vi "Read_Env.vi"(0 "COM Bluegiga in":refnum<visa-resource-name>, 2 "Handle table":string[][](array[string]), 5 "Characteristic UUID":string, 6 "Service UUID":string, 7 "error in (no error)":errorcluster, 15 "Connection Status":T1={"MAC Address"="", "cnx handle"=0, "cnx flags"=0, "Address Type"=125, "Connection Interval (ms)"=125, "Timeout(ms)"=125, "Latency"=0, "bonding handle"=0} {"Address Type" items=["Public", "Random"]}) -> (8 "Intervalo Temperatura":u16, 9 "Intensidad Verde":u8, 10 "Intervalo Humedad":u16, 11 "Intensidad Azul":u8, 12 "Intervalo Presion":u16, 14 "Intervalo Color":u16, 16 "Modo Aire":u8, 18 "Intensidad Rojo":u8, 20 "COM Bluegiga out":refnum<visa-resource-name>, 23 "Registro Completo":u8[](array[numeric]), 27 "error out":errorcluster)   [LabVIEW 2020]
uses:
  <vilib>/BLE/type_def/connection_status_bundle.ctl
  <vilib>/BLE/type_def/address_type.ctl
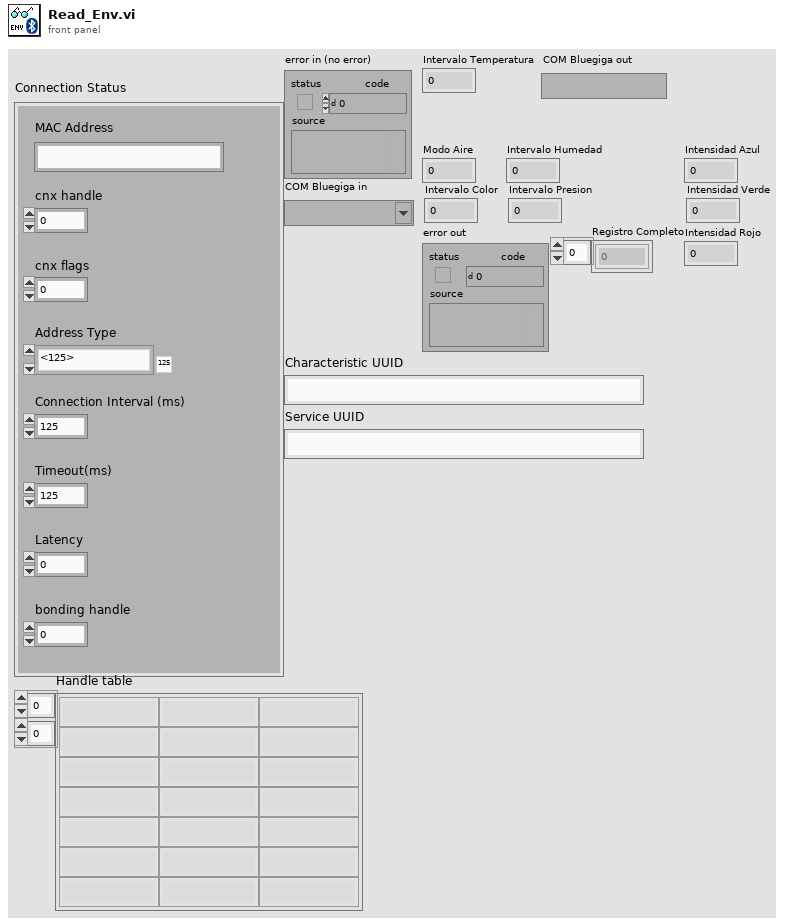
[diagram p1: front panel]
types:
  T1 = typedef "connection_status_bundle.ctl" = cluster{"MAC Address":string, "cnx handle":u8, "cnx flags":u8, "Address Type":T2, "Connection Interval (ms)":u16, "Timeout(ms)":u16, "Latency":u16, "bonding handle":u8}
  T2 = typedef "address_type.ctl" = u8
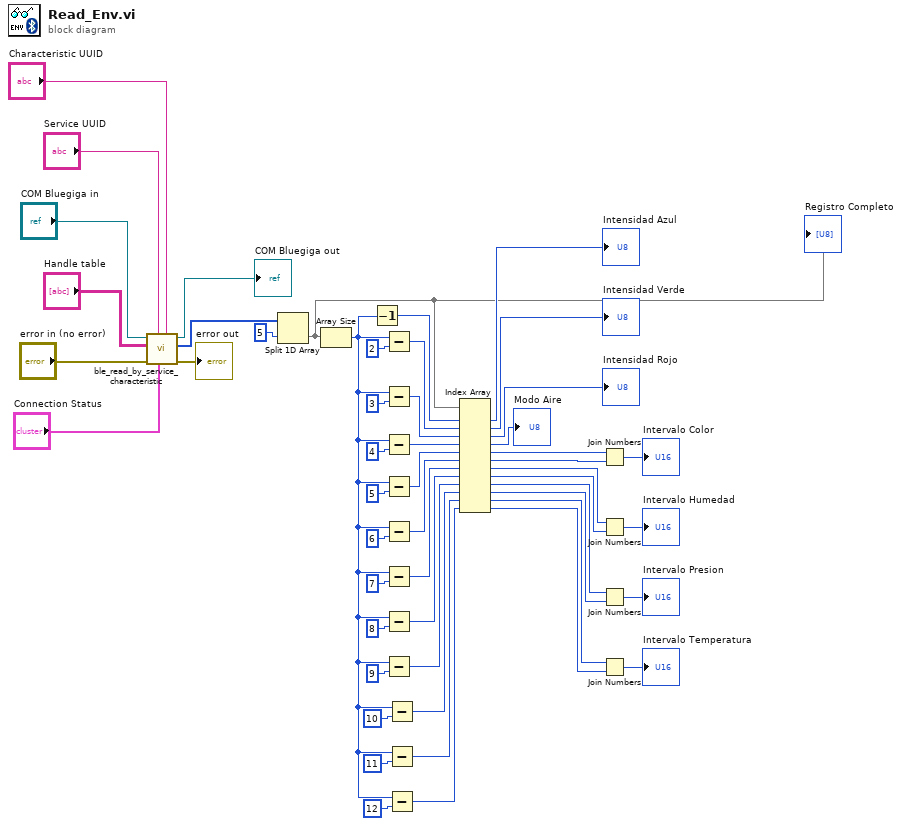
[diagram p0: block diagram]
diagram:
  n1 = call <vilib>:"ble_read_by_service_characteristic.vi"("Characteristic UUID"="Characteristic UUID", "Connection Status"="Connection Status", "Service UUID"="Service UUID", "error in (no error)"="error in (no error)", "Handle table"="Handle table", "COM Bluegiga in"="COM Bluegiga in") -> ("error out"=→"error out":errorcluster, "characteristic value"=w9:u8[], "COM Bluegiga out"=→"COM Bluegiga out":refnum<visa-resource-name>)  [unwired: 3 in]
  n2 = Split 1D Array(array=w9, index=5) -> (second subarray=w11:u8[])  [unwired: 1 out]
  "Registro Completo" <- w11
  n3 = Array Size(array=w11) -> (size(s)=w41:i32)
  n4 = Decrement(x=w41) -> (x-1=w51:i32)
  n5 = Subtract(x=w41, y=2) -> (x-y=w50:i32)
  n6 = Subtract(x=w41, y=3) -> (x-y=w49:i32)
  n7 = Subtract(x=w41, y=4) -> (x-y=w48:i32)
  n8 = Subtract(x=w41, y=5) -> (x-y=w47:i32)
  n9 = Subtract(x=w41, y=6) -> (x-y=w46:i32)
  n10 = Subtract(x=w41, y=7) -> (x-y=w45:i32)
  n11 = Subtract(x=w41, y=8) -> (x-y=w44:i32)
  n12 = Subtract(x=w41, y=9) -> (x-y=w43:i32)
  n13 = Subtract(x=w41, y=10) -> (x-y=w42:i32)
  n14 = Subtract(x=w41, y=11) -> (x-y=w40:i32)
  n15 = Subtract(x=w41, y=12) -> (x-y=w39:i32)
  n16 = Index Array(array=w11, index #1=w51, index #2=w50, index #3=w49, index #4=w48, index #5=w47, index #6=w46, index #7=w45, index #8=w44, index #9=w43, index #10=w42, index #11=w40, index #12=w39) -> (element #1=→"Intensidad Azul":u8, element #2=→"Intensidad Verde":u8, element #3=→"Intensidad Rojo":u8, element #4=→"Modo Aire":u8, element #5=w38:u8, element #6=w37:u8, element #7=w36:u8, element #8=w35:u8, element #9=w34:u8, element #10=w33:u8, element #11=w32:u8, element #12=w31:u8)
  n17 = Join Numbers(hi=w38, lo=w37) -> ((hi.lo)=→"Intervalo Color":u16)
  n18 = Join Numbers(hi=w36, lo=w35) -> ((hi.lo)=→"Intervalo Humedad":u16)
  n19 = Join Numbers(hi=w34, lo=w33) -> ((hi.lo)=→"Intervalo Presion":u16)
  n20 = Join Numbers(hi=w32, lo=w31) -> ((hi.lo)=→"Intervalo Temperatura":u16)
